vi "[CS] [Frame] Threshold.vi"(8 "Threshold":u8, 11 "buffer in":u16[][](array[numeric])) -> (3 "buffer out":u16[][](array[numeric]))   [LabVIEW 2014]
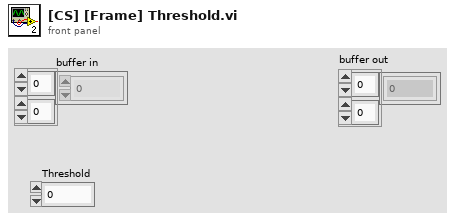
[diagram p1: front panel]
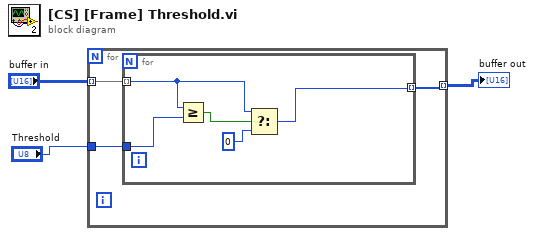
[diagram p0: block diagram]
diagram:
  n1 = for {
    tunnel: "buffer in" -> [w6] mode=indexing
    tunnel: [w5] -> w2 mode=indexing
    tunnel: "Threshold" -> [w4]
    n2 = for {
      tunnel: w6 -> [w9] mode=indexing
      tunnel: [w7] -> w5 mode=indexing
      tunnel: w4 -> [w11]
      n3 = Greater Or Equal?(x=w9, y=w11) -> (x >= y?=w10:bool)
      n4 = Select(t=w9, s=w10, f=u8 0) -> (s? t:f=w7:u16)
    }
  }
  "buffer out" <- w2
